vi "Get_Auth_URL.vi"(8 "error in (no error)":errorcluster, 11 "OneNote in":refnum<class "OneNote.lvclass">) -> (0 "error out":errorcluster, 3 "OneNote out":refnum<class "OneNote.lvclass">)   [LabVIEW 2016, in "OneNote.lvclass"]
uses:
  OneNote.lvclass
  OneNote.lvclass/OneNote.ctl
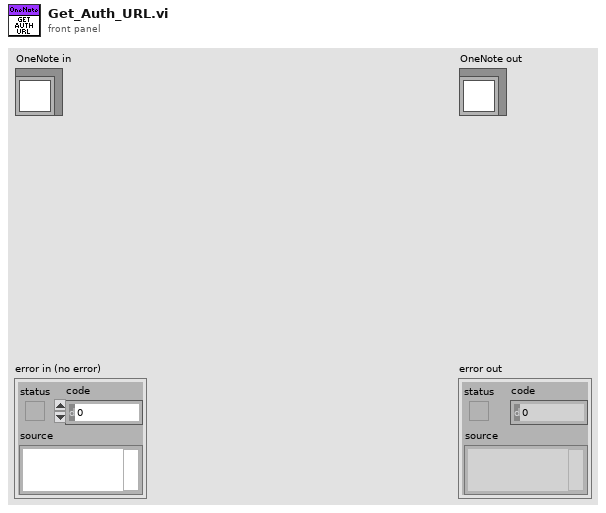
[diagram p1: front panel]
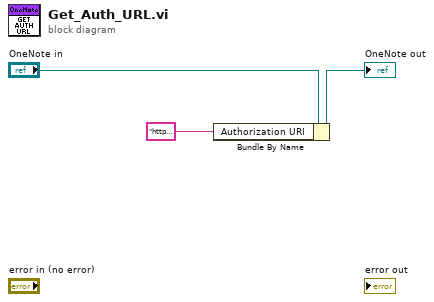
[diagram p0: block diagram]
diagram:
  n1 = Bundle By Name(cluster="OneNote in", "Authorization URI"="https://login.microsoftonline.com/common/oauth2/v2.0/authorize?client_id=e084995a-f38f-442c-a825-de4ec4043537&response_type=code&redirect_uri=https://login.microsoftonline.com/common/oauth2/nativeclient&response_mode=query&scope=User.ReadWrite.All%20offline_access%20Notes.Create%20Notes.ReadWrite.All") -> (→"OneNote out":refnum<class "OneNote.lvclass">)
